vi "ReLu_suv.vi"(1 "Input":dbl) -> (0 "Output":dbl)   [LabVIEW 2021]
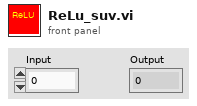
[diagram p1: front panel]
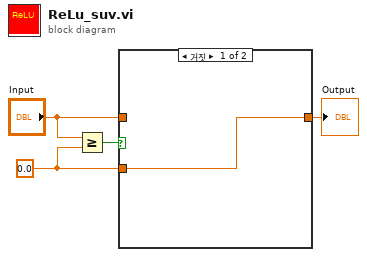
[diagram p0: block diagram]
diagram:
  w1 = 0.0 ("y")
  n1 = Greater Or Equal?(x="Input", y=w1) -> (x >= y?=w4:bool)
  n2 = case shown="거짓" w4 {
    tunnel: [w5 w6] -> w2
    tunnel: "Input" -> [_ w6]
    tunnel: w1 -> [w5 _]
    frame False {
    }
    frame True {
    }
  }
  "Output" <- w2
